vi "Simple ByRef Ex.vi"() -> ()   [LabVIEW 2020]
uses:
  ByRef Example/ByRef Example.lvclass
panel:
  in  "Stop":bool
  out "B":bool
  out "A":bool
  in  "Boolean":bool
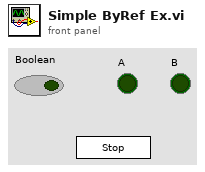
[diagram p1: front panel]
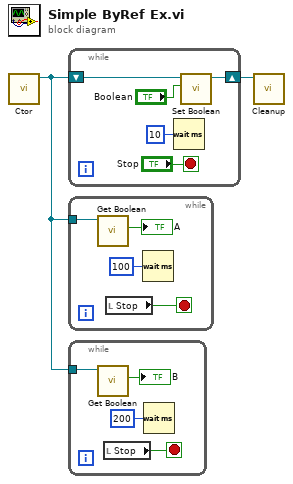
[diagram p0: block diagram]
diagram:
  n1 = call "Ctor.vi"() -> ("ByRef Example out"=w2:refnum<class "ByRef Example.lvclass">)  [unwired: 10 in, 1 out]
  n2 = while {
    shift-right: [w3] -> w1
    shift-left: w2 -> [w7]
    stop <- "Stop" stop-if-true
    n3 = Wait (ms)(milliseconds to wait=u32 10) -> ()  [unwired: 1 out]
    n4 = call "Set Boolean.vi"("Boolean"="Boolean", "ByRef Example in"=w7) -> ("ByRef Example out"=w3:refnum<class "ByRef Example.lvclass">)  [unwired: 8 in, 1 out]
  }
  n5 = while {
    tunnel: w2 -> [w11]
    stop <- w8 stop-if-true
    n6 = call "Get Boolean.vi"("ByRef Example in"=w11) -> ("Boolean"=→"A":bool)  [unwired: 8 in, 2 out]
    n7 = local read "Stop"() -> (w8:bool)
    n8 = Wait (ms)(milliseconds to wait=u32 100) -> ()  [unwired: 1 out]
  }
  n9 = while {
    tunnel: w2 -> [w15]
    stop <- w12 stop-if-true
    n10 = call "Get Boolean.vi"("ByRef Example in"=w15) -> ("Boolean"=→"B":bool)  [unwired: 8 in, 2 out]
    n11 = local read "Stop"() -> (w12:bool)
    n12 = Wait (ms)(milliseconds to wait=u32 200) -> ()  [unwired: 1 out]
  }
  n13 = call "Cleanup.vi"("ByRef Example in"=w1) -> ()  [unwired: 10 in, 1 out]
